vi "DSF.Execution.Runtime.Plugin Manager.Cast Objects.vi"(8 "error in (no error)":errorcluster, 10 "Plugin objects":refnum<class>[](array[class]), 11 "Plugin Manager in":refnum<class "DSF.Engine.Runtime.Plugin Manager.lvclass">) -> (0 "error out":errorcluster, 2 "Plugin":refnum<class "Plugin.lvclass">, 3 "Plugin Manager out":refnum<class "DSF.Engine.Runtime.Plugin Manager.lvclass">)   [LabVIEW 2016, in "DSF.Engine.lvlib" / "DSF.Engine.Runtime.Plugin Manager.lvclass"]
uses:
  DSF.Engine.Runtime.Plugin Manager.lvclass
  Plugin/Plugin.lvclass
  Shared/Typedefs/DSF.Shared.Typedefs.Plugin Classes.ctl
  Shared/Typedefs/DSF.Shared.Typedefs.Plugin Classes.Configuration.ctl
  Shared/Classes/Plugin/DSF.Shared.Configuration.Plugin.lvclass
  Shared/Classes/Transfer Group/DSF.Shared.Configuration.Transfer Group.lvclass
  Shared/Classes/Transfer/DSF.Shared.Configuration.Transfer.lvclass
  Shared/Typedefs/DSF.Shared.Typedefs.Plugin Classes.Runtime.ctl
  Plugin/DSF.Engine.Runtime.Plugin.lvclass
  Shared/Classes/Plugin/DSF.Shared.Runtime.Plugin.Find First Instance.vi
  Shared/Classes/Transfer/DSF.Shared.Configuration.Transfer.Find First Instance.vi
  Shared/Classes/Transfer Group/DSF.Shared.Configuration.Transfer Group.Find First Instance.vi
  Shared/Classes/Plugin/DSF.Shared.Configuration.Plugin.Find First Instance.vi
  DSF.Shared.lvlib
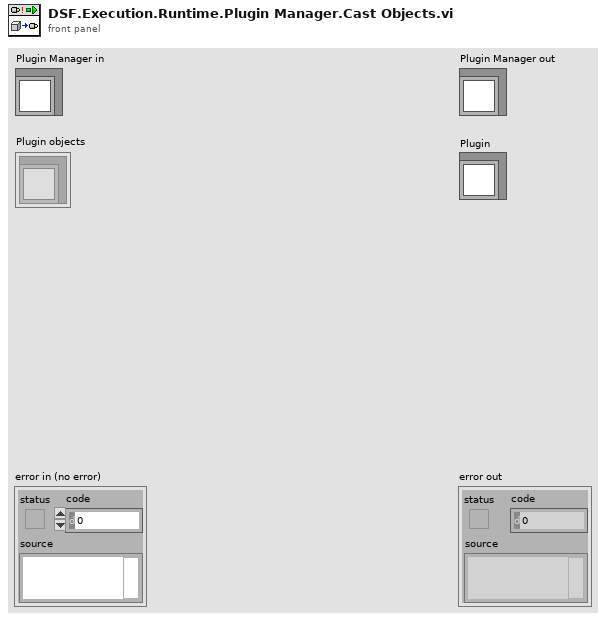
[diagram p1: front panel]
types:
  T1 = typedef "DSF.Shared.lvlib/DSF.Shared.Typedefs.Plugin Classes.ctl" = cluster{"Configuration":T2, "Runtime":T3}
  T2 = typedef "DSF.Shared.lvlib/DSF.Shared.Typedefs.Plugin Classes.Configuration.ctl" = cluster{"Plugin":refnum<class "DSF.Shared.Configuration.Plugin.lvclass">, "Transfer Group":refnum<class "DSF.Shared.Configuration.Transfer Group.lvclass">, "Transfer":refnum<class "DSF.Shared.Configuration.Transfer.lvclass">}
  T3 = typedef "DSF.Shared.lvlib/DSF.Shared.Typedefs.Plugin Classes.Runtime.ctl" = cluster{"Plugin":refnum<class "DSF.Engine.Runtime.Plugin.lvclass">}
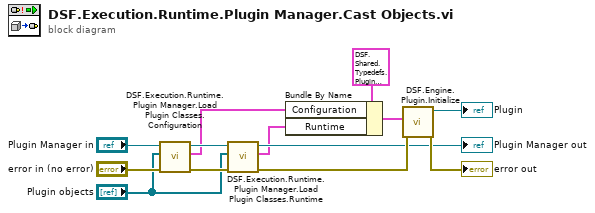
[diagram p0: block diagram]
diagram:
  n1 = call "DSF.Execution.Runtime.Plugin Manager.Load Plugin Classes.Configuration.vi"("error in (no error)"="error in (no error)", "Plugin objects"="Plugin objects", "Plugin Manager in"="Plugin Manager in") -> ("error out"=w10:errorcluster, "Plugin Configuration Classes"=w7:T2, "Plugin Manager out"=w11:refnum<class "DSF.Engine.Runtime.Plugin Manager.lvclass">)  [unwired: 6 in]
  n2 = call "DSF.Execution.Runtime.Plugin Manager.Load Plugin Classes.Runtime.vi"("error in (no error)"=w10, "Plugin objects"="Plugin objects", "Plugin Manager in"=w11) -> ("error out"=w5:errorcluster, "Plugin Runtime Classes"=w1:T3, "Plugin Manager out"=→"Plugin Manager out":refnum<class "DSF.Engine.Runtime.Plugin Manager.lvclass">)  [unwired: 6 in]
  n3 = Bundle By Name(cluster=T1 {"Configuration"={"Plugin"=refnum, "Transfer Group"=refnum, "Transfer"=refnum}, "Runtime"={"Plugin"=refnum}} ("Plugin Classes"), "Configuration"=w7, "Runtime"=w1) -> (w6:T1)
  n4 = call "DSF.Engine.Plugin.Initialize.vi"("error in (no error)"=w5, "Plugin Classes"=w6) -> ("error out"=→"error out":errorcluster, "Plugin out"=→"Plugin":refnum<class "Plugin.lvclass">)  [unwired: 8 in]
